vi "Manager.vi"() -> ()   [LabVIEW 2018]
uses:
  <vilib>/DAQmx/read.llb/DAQmx Read (Digital Bool 1Line 1Point).vi
  <vilib>/DAQmx/write.llb/DAQmx Write (Digital Bool 1Line 1Point).vi
  <vilib>/DAQmx/miscellaneous.llb/DAQmx Fill In Error Info.vi
panel:
  out "data":bool
  in  "data 2":bool
  in  "stop":bool
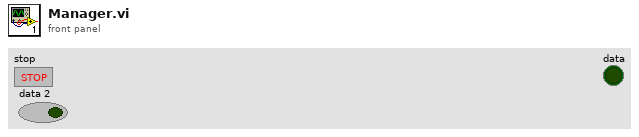
[diagram p1: front panel]
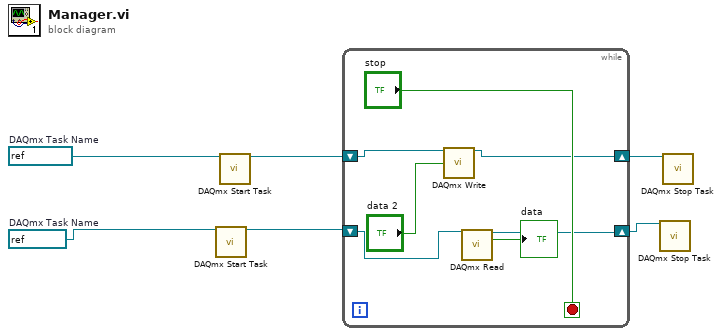
[diagram p0: block diagram]
diagram:
  w3 = refnum<k21> "TEST2"  # DAQmx Task Name
  w4 = refnum<k21> "TEST21"  # DAQmx Task Name
  n1 = call <vilib>:"DAQmx Start Task.vi"("task/channels in"=w3) -> ("task out"=w2:refnum<k21>)  [unwired: 13 in, 1 out]
  n2 = call <vilib>:"DAQmx Start Task.vi"("task/channels in"=w4) -> ("task out"=w6:refnum<k21>)  [unwired: 13 in, 1 out]
  n3 = while {
    shift-right: [w11] -> w5
    shift-left: w6 -> [w12]
    shift-right: [w8] -> w1
    shift-left: w2 -> [w9]
    stop <- "stop" stop-if-true
    n4 = call-poly <vilib>:"DAQmx Write.vi"("task/channels in"=w12, "data"="data 2") -> ("task out"=w11:refnum<k21>)  [unwired: 11 in, 2 out]
    n5 = call-poly <vilib>:"DAQmx Read.vi"("task/channels in"=w9) -> ("task out"=w8:refnum<k21>, "data"=→"data":bool)  [unwired: 12 in, 1 out]
  }
  n6 = call <vilib>:"DAQmx Stop Task.vi"("task/channels in"=w1) -> ()  [unwired: 13 in, 2 out]
  n7 = call <vilib>:"DAQmx Stop Task.vi"("task/channels in"=w5) -> ()  [unwired: 13 in, 2 out]
